vi "Fpga-Top-Level.vi"() -> ()   [LabVIEW 2016]
uses:
  <vilib>/Platform/TimedLoop/XDataNode/timing_clust.ctl
  <vilib>/Platform/TimedLoop/XDataNode/nitl_modes.ctl
  <vilib>/Platform/TimedLoop/XDataNode/wakeup.ctl
  <vilib>/rvi/Emulation/niFpgaSctlEmulationGetInTimedLoop.vi
  <vilib>/rvi/Emulation/niFpgaEmulationReportErrorSimple.vi
  <vilib>/rvi/Emulation/niFpgaGetClockAttributes.vi
  <vilib>/rvi/Emulation/niFpgaCriticalErrorInLSC.vi
  <vilib>/rvi/interface/RandomDataEmulation/niFpgaRandomDataHandleErrors.vi
  <vilib>/Platform/TimedLoop/XDataNode/XDataNode.xnode
  <vilib>/rvi/DataTransferAndStorage/Container/XNode/niFpgaContainer.xnode
  <vilib>/rvi/interface/RandomDataEmulation/nirviRandomDataFpgaReadWriteTemplate.vi
  <vilib>/Platform/TimedLoop/XDataNode/XDNodeRunTimeDep.lvlib
panel:
  out "Seconds":u32 format="%.0x"
  out "MsgType":u8
  out "MsgLen (16)":u16
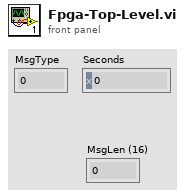
[diagram p1: front panel]
types:
  T1 = typedef "XDNodeRunTimeDep.lvlib/timing_clust.ctl" = cluster{"Expected End [f-1]":u64, "Actual End [f-1]":u64, "Finished Late? [f-1]":bool, "Expected End [i-1]":u64, "Actual End [i-1]":u64, "Finished Late? [i-1]":bool, "Expected Start [i]":u64, "Actual Start [i]":u64, "Expected Start [f]":u64, "Actual Start [f]":u64, "Source Name":string, "Structure Name":string, "Period":i64, "Deadline":i64, "Offset":i64, "Start":i64, "Priority":i32, "Timeout":i32, "Mode":T2, "Wakeup Reason":T3, "Error":errorcluster, "Source Type":string, "Secondary Source Type":string, "Global End Time":u64, "Global Start Time":u64, "Frame Duration":u64, "Iteration Duration":u64, "Assigned CPU":i32, "I/O Scan Engine Mode":u32}
  T2 = typedef "XDNodeRunTimeDep.lvlib/nitl_modes.ctl" = enum32{"No Change", "Process missed periods, maintain original phase", "Discard missed periods, maintain original phase", "Process missed periods, ignore original phase", "Discard missed periods, ignore original phase"}
  T3 = typedef "XDNodeRunTimeDep.lvlib/wakeup.ctl" = enum32{"Normal", "Aborted", "Asynchronous wakeup", "Timing source error", "Timed loop error", "Timeout"}
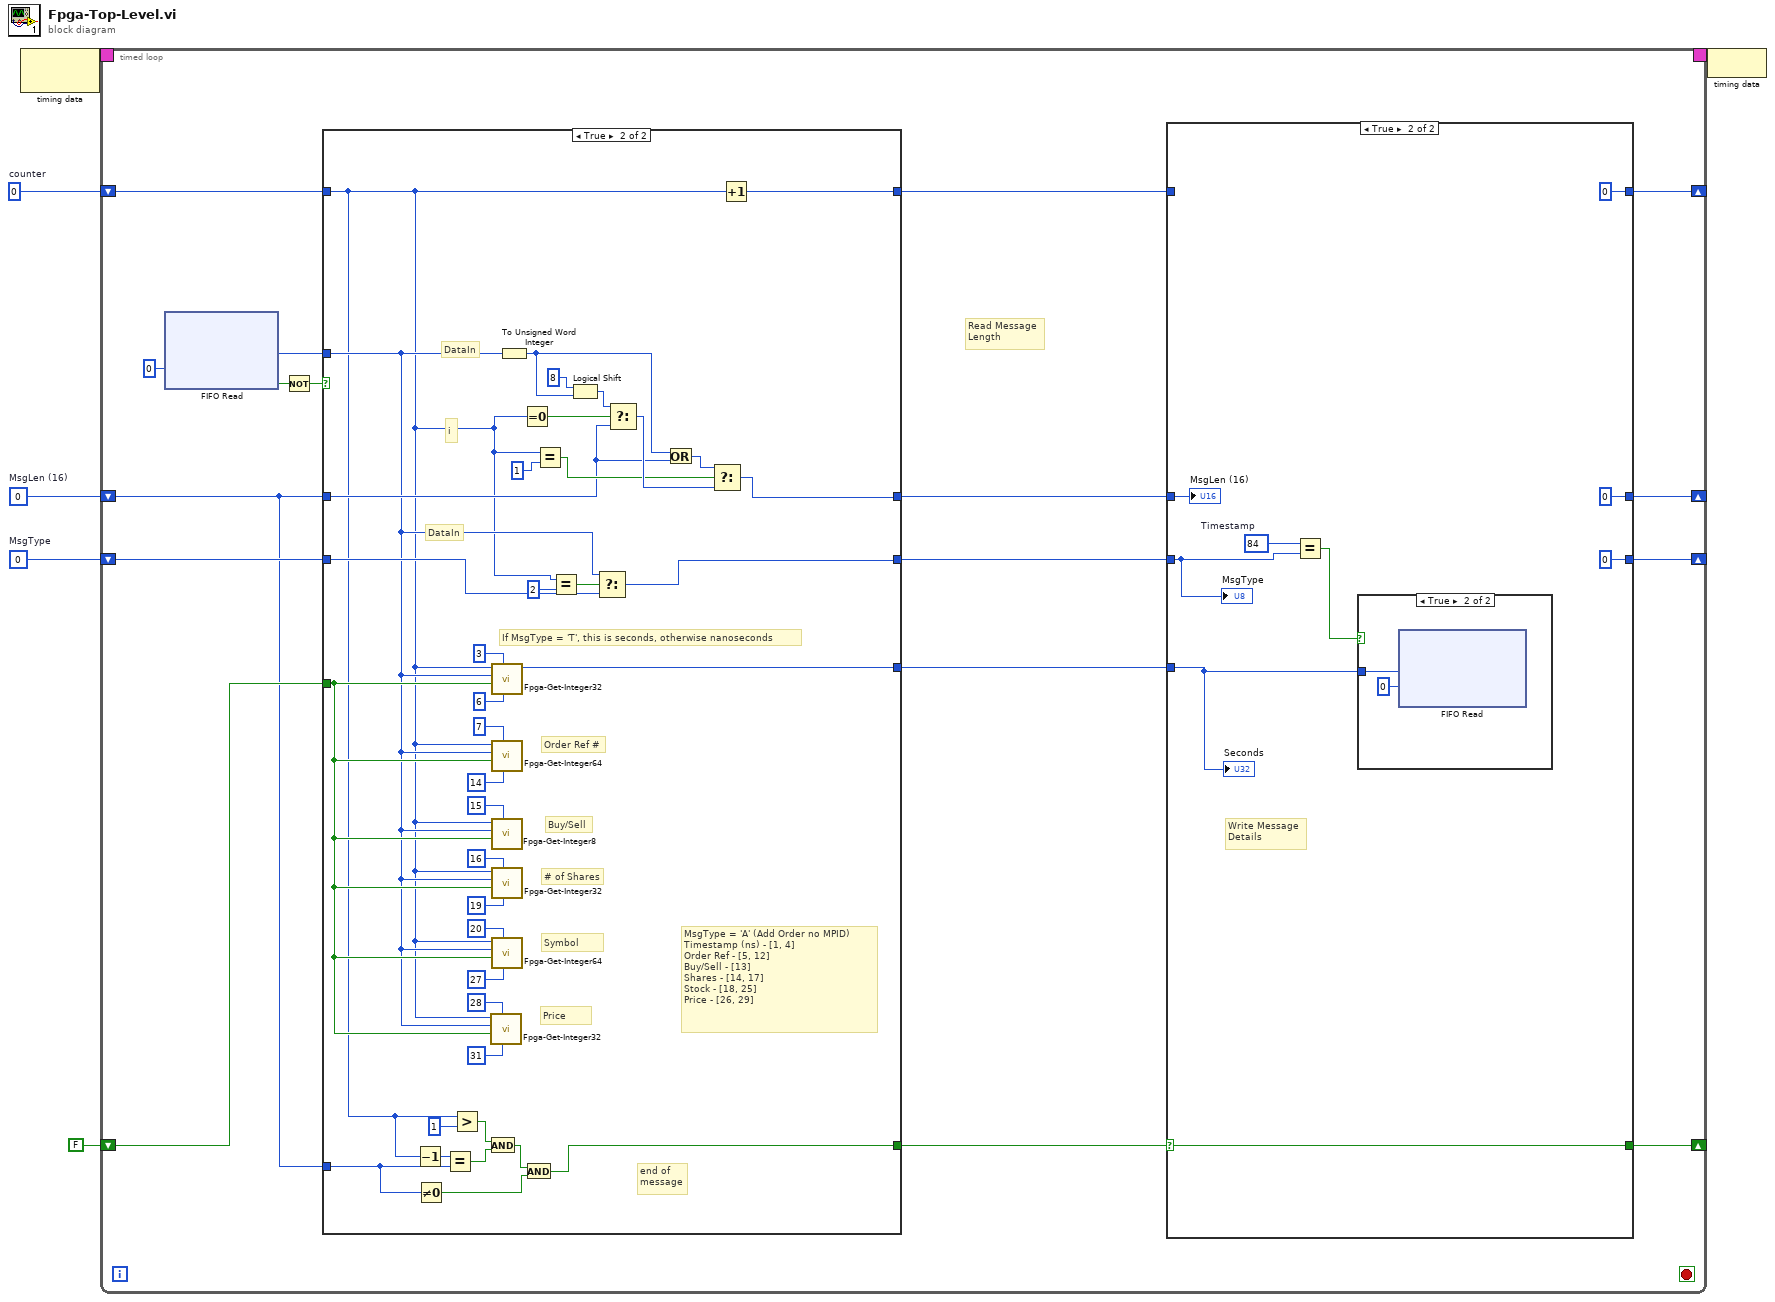
[diagram p0: block diagram]
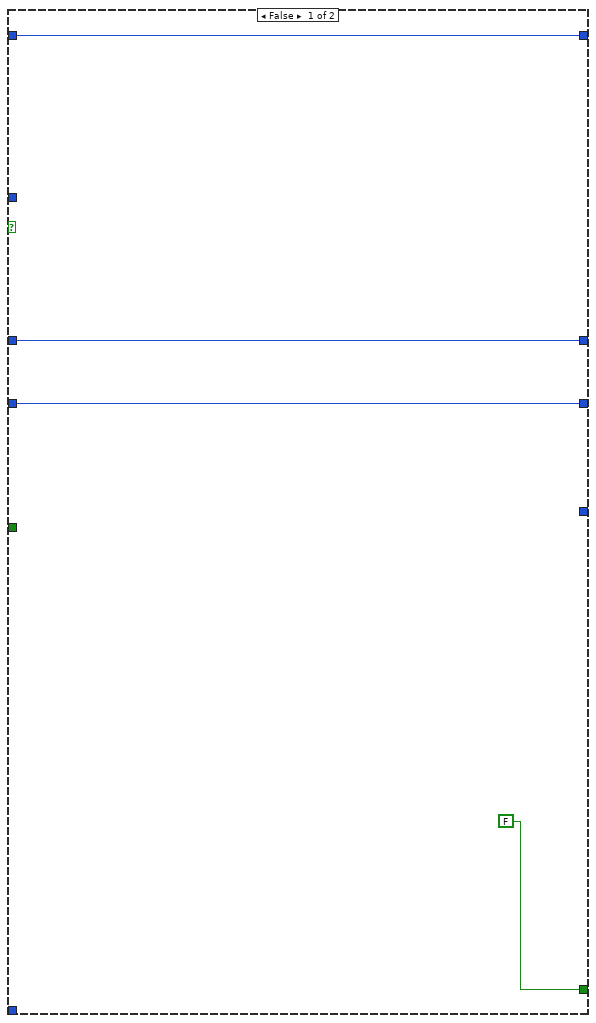
[diagram p4: hidden frame]
diagram:
  w2 = u8 0  # MsgType
  w3 = u16 0  # counter
  w4 = u16 0  # MsgLen (16)
  n1 = node-c288() -> (w6:T1)  [unwired: 1 in]
  n2 = timed-loop {
    timing: w6 -> [_]
    timing-out: [_] -> w5
    shift-right: [w14] -> _
    shift-left: w4 -> [w7]
    shift-right: [w15] -> _
    shift-left: w3 -> [w19]
    shift-right: [w12] -> _
    shift-left: w2 -> [w18]
    shift-right: [w9] -> _
    shift-left: FALSE -> [w8]
    stop <- _ stop-if-true
    # "Read Message\nLength"
    n3 = xnode ("FIFO Read")("Timeout"=0) -> ("Element"=w20:u8, "Timed Out?"=w22:bool)  [unwired: 1 in, 1 out]
    n4 = Not(x=w22) -> (.not. x?=w21:bool)
    n5 = case shown="True" w21 {
      tunnel: w20 -> [_ w53]
      tunnel: [w42 w75] -> w13
      tunnel: w7 -> [w42 w56]
      tunnel: w19 -> [w41 w52]
      tunnel: [w41 w79] -> w16
      tunnel: w18 -> [w40 w65]
      tunnel: [w40 w63] -> w11
      tunnel: [_ w59] -> w10
      tunnel: [FALSE w60] -> w17
      tunnel: w8 -> [_ w54]
      tunnel: w7 -> [_ w55]
      frame False {
      }
      frame True {
        # "MsgType = 'A' (Add Order no MPID)\nTimestamp (ns) - [1, 4]\nOrder Ref - [5, 12]\nBuy/Sell - [13]\nShares - [14, 17]\nStock - [18, 25]\nPrice - [26, 29]"
        # "Buy/Sell"
        # "Order Ref #"
        # "# of Shares"
        # "Symbol"
        # "Price"
        # "If MsgType = 'T', this is seconds, otherwise nanoseconds"
        # "DataIn"
        # "i"
        # "DataIn"
        # "end of\nmessage"
        n6 = Decrement(x=w52) -> (x-1=w67:u16)
        n7 = Not Equal To 0?(x=w55) -> (x != 0?=w62:bool)
        n8 = Equal?(x=w67, y=w55) -> (x = y?=w68:bool)
        n9 = Greater?(x=w52, y=u16 1) -> (0:w69:bool)
        n10 = And(x=w69, y=w68) -> (x .and. y?=w61:bool)
        n11 = call "Fpga-Get-Integer32.vi"("upper"=u16 31 ("lower"), "lower"=u16 28, "Reset"=w54, "DataIn"=w53, "Index"=w52) -> ()  [unwired: 5 in, 2 out]
        n12 = call "Fpga-Get-Integer32.vi"("upper"=u16 6, "lower"=u16 3, "Reset"=w54, "DataIn"=w53, "Index"=w52) -> ("UInt32"=w59:u32)  [unwired: 5 in, 1 out]
        n13 = call "Fpga-Get-Integer64.vi"("upper"=u16 14 ("lower"), "lower"=u16 7, "Reset"=w54, "DataIn"=w53, "Index"=w52) -> ()  [unwired: 5 in, 2 out]
        n14 = call "Fpga-Get-Integer8.vi"("lower"=u16 15, "Reset"=w54, "DataIn"=w53, "Index"=w52) -> ()  [unwired: 6 in, 2 out]
        n15 = call "Fpga-Get-Integer32.vi"("upper"=u16 19 ("lower"), "lower"=u16 16, "Reset"=w54, "DataIn"=w53, "Index"=w52) -> ()  [unwired: 5 in, 2 out]
        n16 = call "Fpga-Get-Integer64.vi"("upper"=u16 27 ("lower"), "lower"=u16 20, "Reset"=w54, "DataIn"=w53, "Index"=w52) -> ()  [unwired: 5 in, 2 out]
        n17 = To Unsigned Word Integer(number=w53) -> (unsigned 16bit integer=w71:u16)
        n18 = Equal To 0?(x=w52) -> (x = 0?=w78:bool)
        n19 = And(x=w61, y=w62) -> (x .and. y?=w60:bool)
        n20 = Equal?(x=w52, y=u16 1) -> (x = y?=w76:bool)
        n21 = Equal?(x=w52, y=u16 2) -> (x = y?=w64:bool)
        n22 = Logical Shift(y=i16 8, x=w71) -> (x << y=w72:u16)
        n23 = Select(t=w53, s=w64, f=w65) -> (s? t:f=w63:u8)
        n24 = Select(t=w72, s=w78, f=w56) -> (s? t:f=w77:u16)
        n25 = Or(x=w71, y=w56) -> (x .or. y?=w74:u16)
        n26 = Select(t=w74, s=w76, f=w77) -> (s? t:f=w75:u16)
        n27 = Increment(x=w52) -> (x+1=w79:u16)
      }
    }
    n28 = case shown="True" w17 {
      selector: w17 -> [w24 w28]
      tunnel: w16 -> [w25 _]
      tunnel: [w25 u16 0 ("counter")] -> w15
      tunnel: [w26 u16 0 ("MsgLen (16)")] -> w14
      tunnel: w13 -> [w26 w36]
      tunnel: [w27 u8 0 ("MsgType")] -> w12
      tunnel: w11 -> [w27 w31]
      tunnel: w10 -> [_ w35]
      tunnel: [w24 w28] -> w9
      frame False {
      }
      frame True {
        w30 = u8 84  # Timestamp
        # "Write Message\nDetails"
        n29 = Equal?(x=w30, y=w31) -> (x = y?=w29:bool)
        n30 = case shown="True" w29 {
          tunnel: w35 -> [_ w37]
          frame False {
          }
          frame True {
            n31 = xnode ("FIFO Read")("Element"=w37, "Timeout"=0) -> ()  [unwired: 1 in, 2 out]
          }
        }
        "MsgLen (16)" <- w36
        "MsgType" <- w31
        "Seconds" <- w35
      }
    }
  }
  n32 = node-c288(w5) -> ()
